vi "DCA Harvest Units from Name.vi"(2 "Name (Units)":string) -> (6 "Name":string, 7 "Units":string)   [LabVIEW 2011]
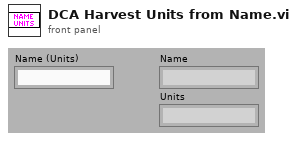
[diagram p1: front panel]
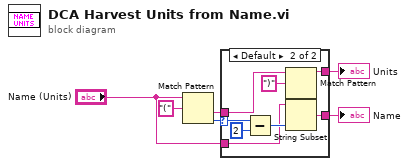
[diagram p0: block diagram]
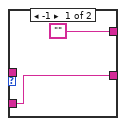
[diagram p2: hidden frame]
diagram:
  n1 = Match Pattern(string="Name (Units)", regular expression="(") -> (after substring=w3:string, offset past match=w1:i32)  [unwired: 3 out]
  n2 = case shown="Default" w1 {
    selector: w1 -> [_ w9]
    tunnel: [w8 w13] -> w5
    tunnel: ["" w12] -> w4
    tunnel: w3 -> [_ w11]
    tunnel: "Name (Units)" -> [w8 w10]
    frame -1 {
    }
    frame Default {
      n3 = Subtract(x=w9, y=2) -> (x-y=w15:i32)
      n4 = Match Pattern(string=w11, regular expression=")") -> (before substring=w12:string)  [unwired: 4 out]
      n5 = String Subset(string=w10, length (rest)=w15) -> (substring=w13:string)  [unwired: 1 out]
    }
  }
  "Name" <- w5
  "Units" <- w4
